vi "oax_Tacho Channel Warning (DSA).vi"(8 "error in (no error)":errorcluster, 11 "legal channels":tag[](array[tag])) -> (0 "error out":errorcluster, 2 "tacho channel index":i32, 3 "tachometer channel":tag)   [LabVIEW 2017]
panel:
  in  "tachometer channel":u16(ring) items=["Dev3/ai0"]
  in  "Stop":bool
  # "Incorrect tachometer channel selection!"
  # "The tachometer channel is not selected in Channels selection"
  # "Select the correct tachometer channel:"
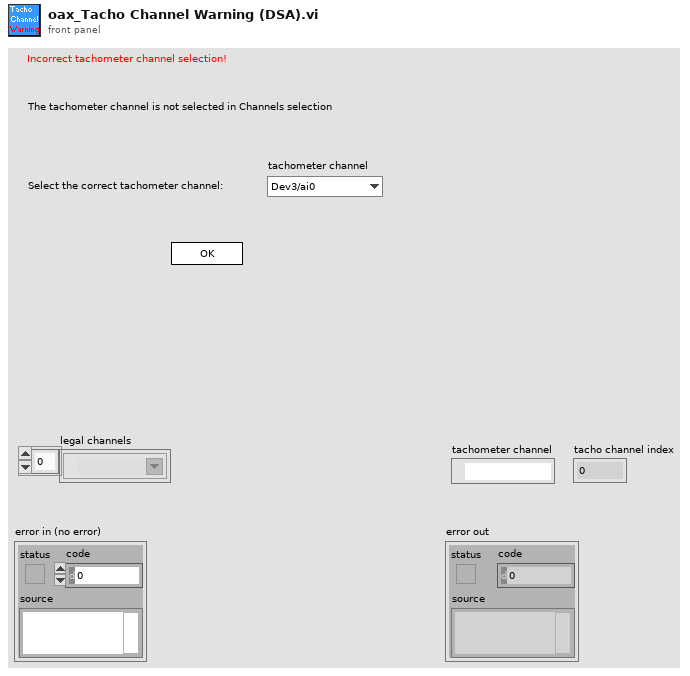
[diagram p1: front panel]
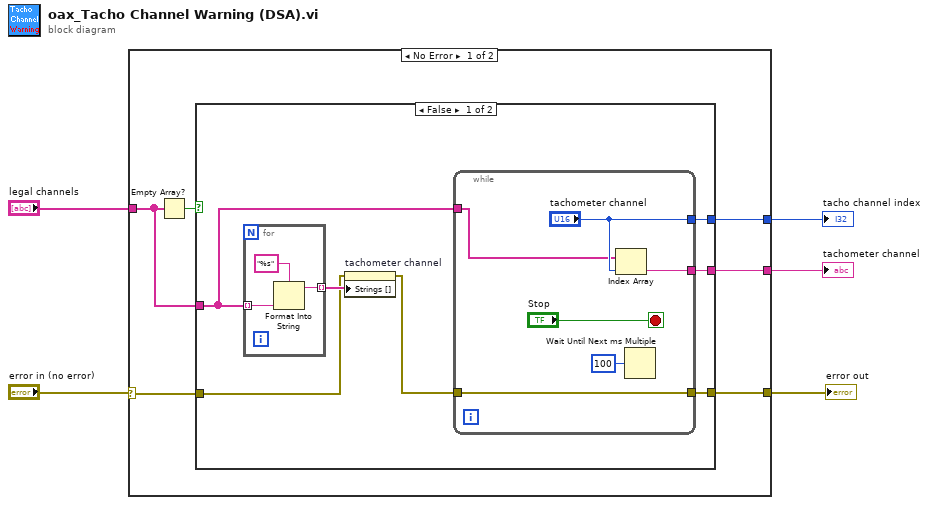
[diagram p0: block diagram]
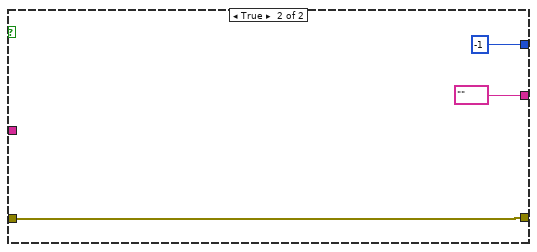
[diagram p2: hidden frame]
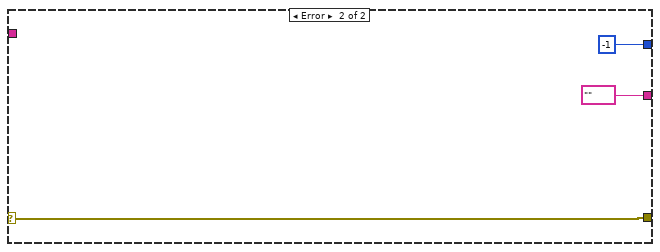
[diagram p3: hidden frame]
diagram:
  n1 = case shown="No Error" "error in (no error)" {
    selector: "error in (no error)" -> [w9 w31]
    tunnel: [w11 w31] -> w5
    tunnel: "legal channels" -> [w10 _]
    tunnel: [w7 -1 ("tacho channel index")] -> w2
    tunnel: [w6 tag "" ("tachometer channel")] -> w1
    frame No Error {
      n2 = Empty Array?(array=w10) -> (empty?=w8:bool)
      n3 = case shown="False" w8 {
        tunnel: [w18 w28] -> w11
        tunnel: w10 -> [w14 _]
        tunnel: w9 -> [w15 w28]
        tunnel: [w13 -1 ("tacho channel index")] -> w7
        tunnel: [w12 tag "" ("tachometer channel")] -> w6
        frame False {
          n4 = for {
            tunnel: w14 -> [w19] mode=indexing
            tunnel: [w20] -> w17 mode=indexing
            n5 = Format Into String(format string="%s", w19) -> (resulting string=w20:string)  [unwired: 2 in, 1 out]
          }
          n6 = property on="tachometer channel" class="Ring (strict)"(error in=w15, "Strings []"=w17) -> (error out=w16:errorcluster)  [unwired: 1 in, 1 out]
          n7 = while {
            tunnel: w16 -> [w27]
            tunnel: [w27] -> w18
            tunnel: w14 -> [w23]
            tunnel: ["tachometer channel"] -> w13
            tunnel: [w22] -> w12
            stop <- "Stop" stop-if-true
            n8 = Index Array(array=w23, index="tachometer channel") -> (element=w22:tag)
            n9 = Wait Until Next ms Multiple(millisecond multiple=u32 100) -> ()  [unwired: 1 out]
          }
        }
        frame True {
        }
      }
    }
    frame Error {
    }
  }
  "error out" <- w5
  "tachometer channel" <- w1
  "tacho channel index" <- w2
